vi "SMT_Read.vi"(0 "Traceability 引用句柄":refnum<k24>, 1 "Type":string, 2 "Status":string, 3 "EndDate":string, 5 "LoadID":string, 7 "ItemID":string, 9 "CellID":string, 11 "error in (no error)":errorcluster caption="错误输入（无错误）", 12 "History":i32, 13 "StartDate":string, 14 "tblName":string) -> (4 "Traceability 引用句柄输出":refnum<k24>, 6 ".NET:System.Data.DataSet":T1={"CaseSensitive"=FALSE, "Container"=refnum, "DataSetName"="", "DefaultViewManager"=refnum, "DesignMode"=FALSE, "EnforceConstraints"=FALSE, "ExtendedProperties"=refnum, "HasErrors"=FALSE, "IsInitialized"=FALSE, "Locale"=refnum, "Namespace"="", "Prefix"="", "Relations"=refnum, "RemotingFormat"=0, "SchemaSerializationMode"=1, "Site"=refnum, "Tables"=refnum} {"SchemaSerializationMode" items=["IncludeSchema"=1, "ExcludeSchema"=2]; "RemotingFormat" items=["Xml", "Binary"]}, 15 "error out":errorcluster caption="错误输出")   [LabVIEW 2014, in "Traceability.lvlib"]
uses:
  D:/webservice/Traceability.dll
  Traceability.dll
  System.Data
  Traceability.lvlib
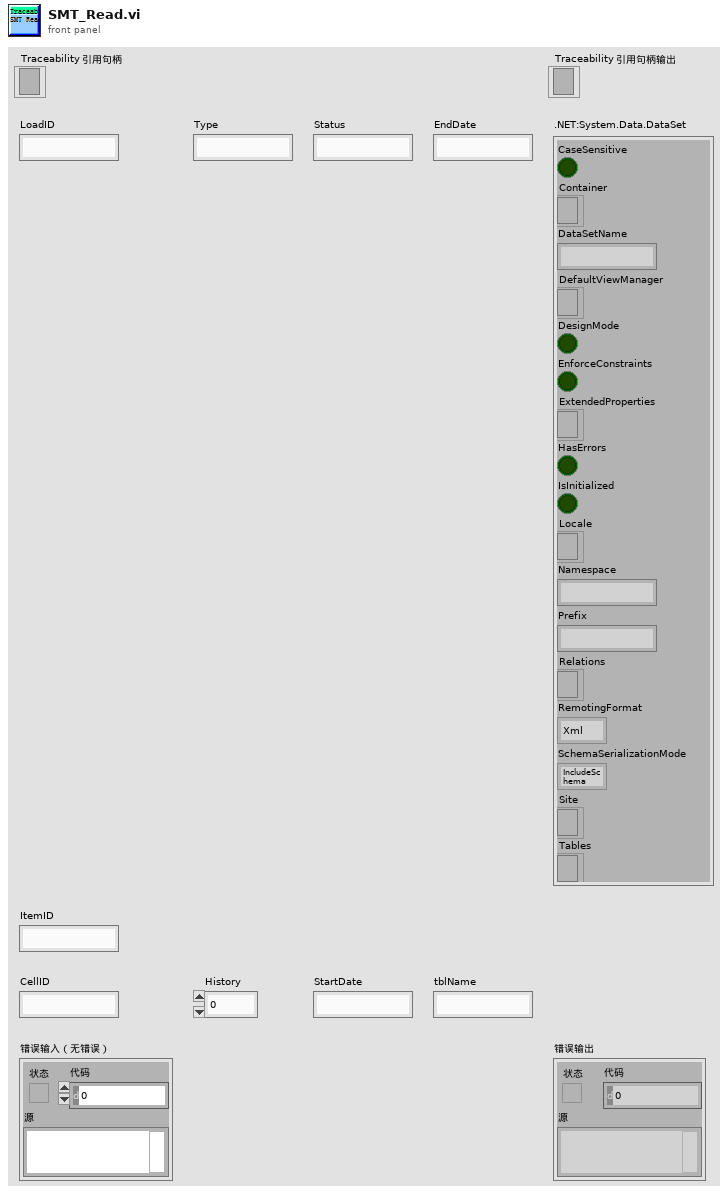
[diagram p1: front panel]
types:
  T1 = cluster{"CaseSensitive":bool, "Container":refnum<k24>, "DataSetName":string, "DefaultViewManager":refnum<k24>, "DesignMode":bool, "EnforceConstraints":bool, "ExtendedProperties":refnum<k24>, "HasErrors":bool, "IsInitialized":bool, "Locale":refnum<k24>, "Namespace":string, "Prefix":string, "Relations":refnum<k24>, "RemotingFormat":i32, "SchemaSerializationMode":i32, "Site":refnum<k24>, "Tables":refnum<k24>}
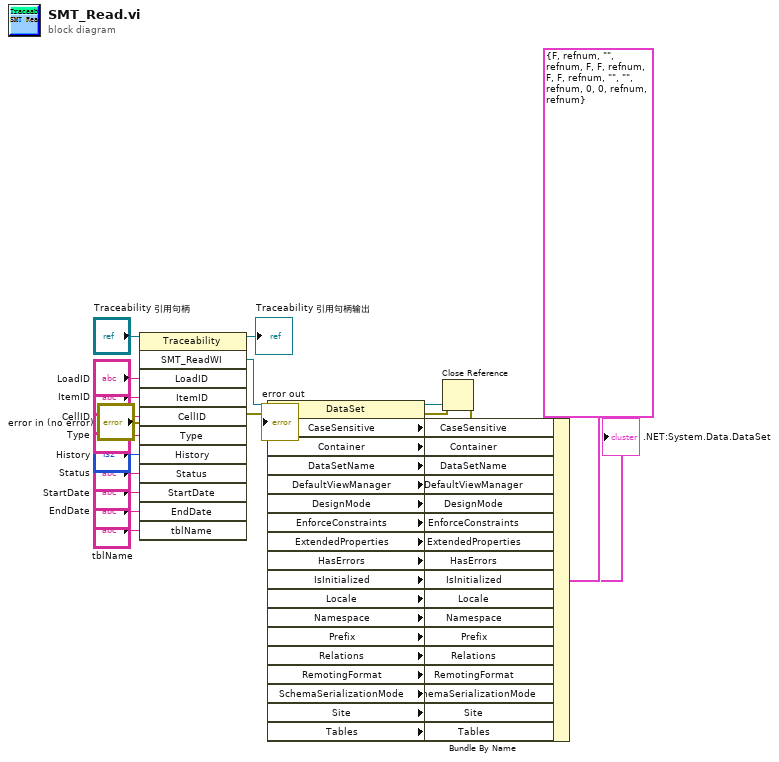
[diagram p0: block diagram]
diagram:
  n1 = invoke class="Traceability" method="SMT_ReadWI"(reference="Traceability 引用句柄", error in="error in (no error)", "LoadID"="LoadID", "ItemID"="ItemID", "CellID"="CellID", "Type"="Type", "History"="History", "Status"="Status", "StartDate"="StartDate", "EndDate"="EndDate", "tblName"="tblName") -> (reference out=→"Traceability 引用句柄输出":refnum<k24>, error out=w4:errorcluster, "SMT_ReadWI"=w33:refnum<k24>)  [unwired: 1 in, 9 out]
  n2 = property class="DataSet"(reference=w33, error in=w4) -> (reference out=w3:refnum<k24>, error out=w2:errorcluster, "CaseSensitive"=w30:bool, "Container"=w29:refnum<k24>, "DataSetName"=w28:string, "DefaultViewManager"=w27:refnum<k24>, "DesignMode"=w26:bool, "EnforceConstraints"=w25:bool, "ExtendedProperties"=w24:refnum<k24>, "HasErrors"=w23:bool, "IsInitialized"=w22:bool, "Locale"=w21:refnum<k24>, "Namespace"=w20:string, "Prefix"=w19:string, "Relations"=w18:refnum<k24>, "RemotingFormat"=w17:i32, "SchemaSerializationMode"=w16:i32, "Site"=w15:refnum<k24>, "Tables"=w14:refnum<k24>)
  n3 = Bundle By Name(cluster=T1 {"CaseSensitive"=FALSE, "Container"=refnum, "DataSetName"="", "DefaultViewManager"=refnum, "DesignMode"=FALSE, "EnforceConstraints"=FALSE, "ExtendedProperties"=refnum, "HasErrors"=FALSE, "IsInitialized"=FALSE, "Locale"=refnum, "Namespace"="", "Prefix"="", "Relations"=refnum, "RemotingFormat"=0, "SchemaSerializationMode"=0, "Site"=refnum, "Tables"=refnum} (".NET:System.Data.DataSet"), "CaseSensitive"=w30, "Container"=w29, "DataSetName"=w28, "DefaultViewManager"=w27, "DesignMode"=w26, "EnforceConstraints"=w25, "ExtendedProperties"=w24, "HasErrors"=w23, "IsInitialized"=w22, "Locale"=w21, "Namespace"=w20, "Prefix"=w19, "Relations"=w18, "RemotingFormat"=w17, "SchemaSerializationMode"=w16, "Site"=w15, "Tables"=w14) -> (→".NET:System.Data.DataSet":T1)
  n4 = Close Reference(reference=w3, error in (no error)=w2) -> (error out=→"error out":errorcluster)
